vi "dsyrk - Symmetric Matrix Rank-k Update (DBL).vi"(4 "beta":dbl=1.0, 6 "alpha":dbl=1.0, 7 "operation A":T1 items=["Direct", "Conjugated & Transposed", "Transposed"], 8 "matrix C type":T2=3 items=["Lower Triangular"=2, "Upper Triangular"=3], 9 "C":T3, 11 "A":T3) -> (0 "error":i32, 3 "dsyrk":T3)   [LabVIEW 2020, in "NI_AALBLAS.lvlib"]
doc: "Calculates the rank-k update of the upper or lower triangular component of a symmetric matrix."
uses:
  NI_AALBLAS.lvlib
  RealMatrix.ctl
  LV_UpLo.ctl
  LV_Transpose.ctl
  Fucntion.ctl
  Order.ctl
  NI_Matrix.lvlib
panel:
  # "dsyrk=alpha*A*A'+beta*C / dsyrk=alpha*A'*A+beta*C"
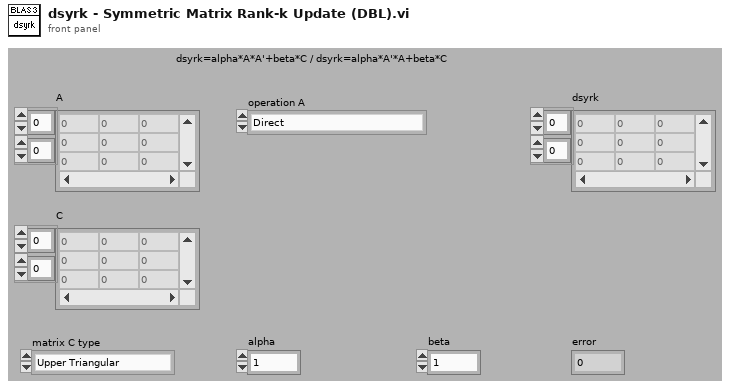
[diagram p1: front panel]
types:
  T1 = typedef "NI_AALBLAS.lvlib/LV_Transpose.ctl" = i32
  T2 = typedef "NI_AALBLAS.lvlib/LV_UpLo.ctl" = i32
  T3 = typedef "NI_Matrix.lvlib/RealMatrix.ctl" = dbl[][]
  T4 = typedef "NI_AALBLAS.lvlib/Order.ctl" = i32
  T5 = typedef "NI_AALBLAS.lvlib/Fucntion.ctl" = u16
  T6 = typedef "NI_AALBLAS.lvlib/Operation_Transpose.ctl" = i32
  T7 = typedef "NI_AALBLAS.lvlib/UpLo.ctl" = i32
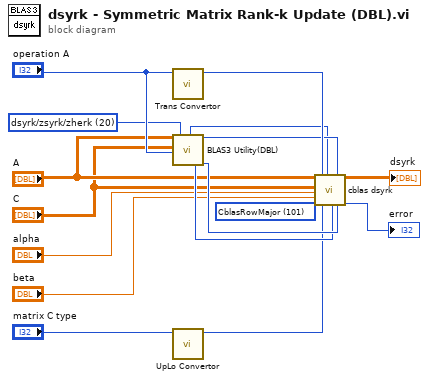
[diagram p0: block diagram]
diagram:
  w1 = T4 101 items=["CblasRowMajor"=101, "CblasColMajor"=102] ("order")
  w2 = T5 20 items=["ddot/zdotu/zdotc", "daxpy/zaxpy", "dnrm2/dznrm2", "dasum/dzasum", "dcopy/zcopy", "dswap/zswap", "drotm", "drot/zdrot", "idamax/izamax", "idamin/izamin", "dgemv/zgemv", "dsymv/zhemv", "dtrmv/ztrmv", "dsyr/zher", "dsyr2/zher2", "dger/zgeru/zgerc", "dtrsv/ztrsv", "dgemm/zgemm", "dsymm/zsymm/zhemm", "dtrmm/ztrmm", "dsyrk/zsyrk/zherk", "dsyr2k/zsyr2k/zher2k", "dtrsm/ztrsm"] ("function")
  n1 = call "Trans Convertor.vi"("operation"="operation A") -> ("trans"=w11:T6)  [unwired: 10 out]
  n2 = call "BLAS3 Utility(DBL).vi"("A"="A", "C"="C", "operation A"="operation A", "function"=w2) -> ("lda"=w3:i32, "n"=w14:i32, "ldc"=w4:i32, "k"=w15:i32)  [unwired: 10 in, 2 out]
  n3 = call "UpLo Convertor.vi"("triangle matrix type"="matrix C type") -> ("uplo"=w9:T7)  [unwired: 10 out]
  n4 = call "cblas dsyrk.vi"("A"="A", "C"="C", "alpha"="alpha", "beta"="beta", "order"=w1, "transA"=w11, "uplo"=w9, "lda"=w3, "n"=w14, "ldc"=w4, "k"=w15) -> ("dsyrk"=→"dsyrk":T3, "error"=→"error":i32)  [unwired: 7 out]
